vi "Destroy Interface.vi"(8 "error in (no error)":errorcluster, 11 "Interface in":refnum<class "Interface.lvclass">) -> (0 "error out":errorcluster, 3 "Interface out":refnum<class "Interface.lvclass">)   [LabVIEW 2019, in "DSF Core.lvlib" / "Interface.lvclass"]
uses:
  Interface.lvclass
  Interface.lvclass/Interface.ctl
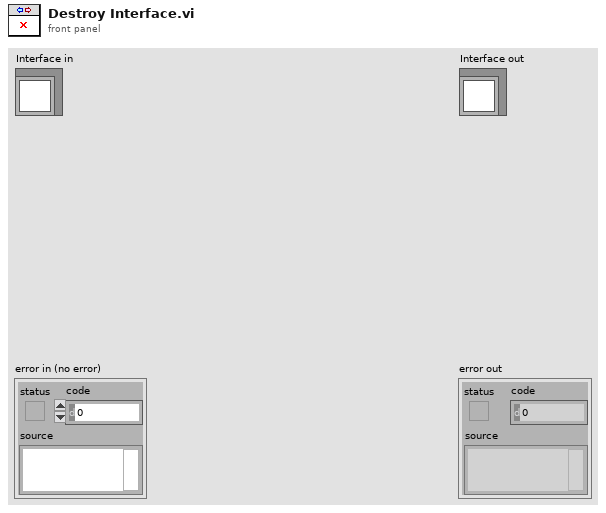
[diagram p1: front panel]
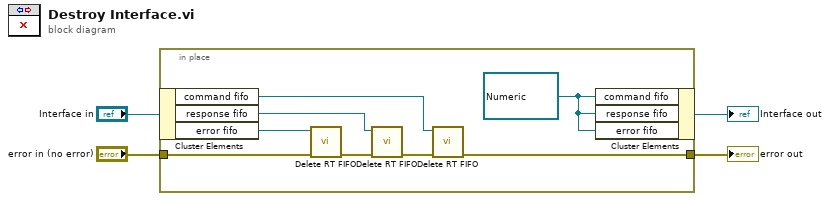
[diagram p0: block diagram]
diagram:
  n1 = in-place {
    in-place-border: "error in (no error)" -> [w12]
    in-place-border: [w6] -> w2
    w5 = refnum<k33> refnum ("Command FIFO")
    n2 = in-place-cluster #1("Interface in") -> ("command fifo"=w7:refnum<k33>, "response fifo"=w8:refnum<k33>, "error fifo"=w9:refnum<k33>)
    n3 = call "Delete RT FIFO.vi"("error in (no error)"=w12, "rt fifo"=w9) -> ("error out"=w11:errorcluster)  [unwired: 9 in]
    n4 = call "Delete RT FIFO.vi"("error in (no error)"=w11, "rt fifo"=w8) -> ("error out"=w10:errorcluster)  [unwired: 9 in]
    n5 = call "Delete RT FIFO.vi"("error in (no error)"=w10, "rt fifo"=w7) -> ("error out"=w6:errorcluster)  [unwired: 9 in]
    n6 = in-place-cluster #1("command fifo"=w5, "response fifo"=w5, "error fifo"=w5) -> (→"Interface out":refnum<class "Interface.lvclass">)
  }
  "error out" <- w2
